vi "Inst_DS360.vi"(8 "error in":errorcluster, 10 "All Message Queues in":T1, 11 "Prueba09 in":refnum<class "Prueba09.lvclass">) -> (0 "error out":errorcluster)   [LabVIEW 2019, in "Prueba09.lvclass"]
uses:
  Prueba09.lvclass
  QMH/Message Queue/All Message Queues.ctl
  QMH/Message Queue/Message Cluster.ctl
  Prueba09.lvclass/Prueba09.ctl
  ClusterGEN.ctl
  <vilib>/Utility/error.llb/Error Cluster From Error Code.vi
  QMH/Message Queue/Enqueue Message (Single).vi
  <vilib>/ErrorRing/Error Ring.xnode
  QMH/Message Queue/Message Queue.lvlib
  Instrumento/DS360/DS360.lvclass
panel:
  out "All States":string[](array[string])
  out "Actual State":string
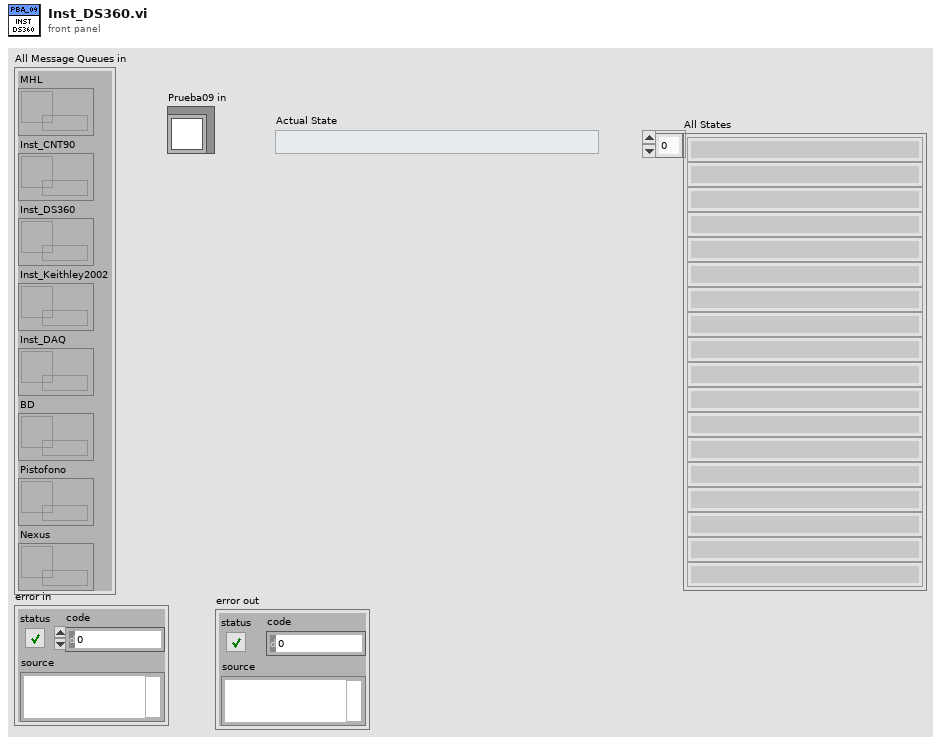
[diagram p1: front panel]
types:
  T1 = typedef "Message Queue.lvlib/All Message Queues.ctl" = cluster{"MHL":refnum<queue>, "Inst_CNT90":refnum<queue>, "Inst_DS360":refnum<queue>, "Inst_Keithley2002":refnum<queue>, "Inst_DAQ":refnum<queue>, "BD":refnum<queue>, "Pistofono":refnum<queue>, "Nexus":refnum<queue>}
  T2 = typedef "Prueba09.lvclass/ClusterGEN.ctl" = cluster{"frec":dbl, "amp":dbl, "tipo_ciclo":string}
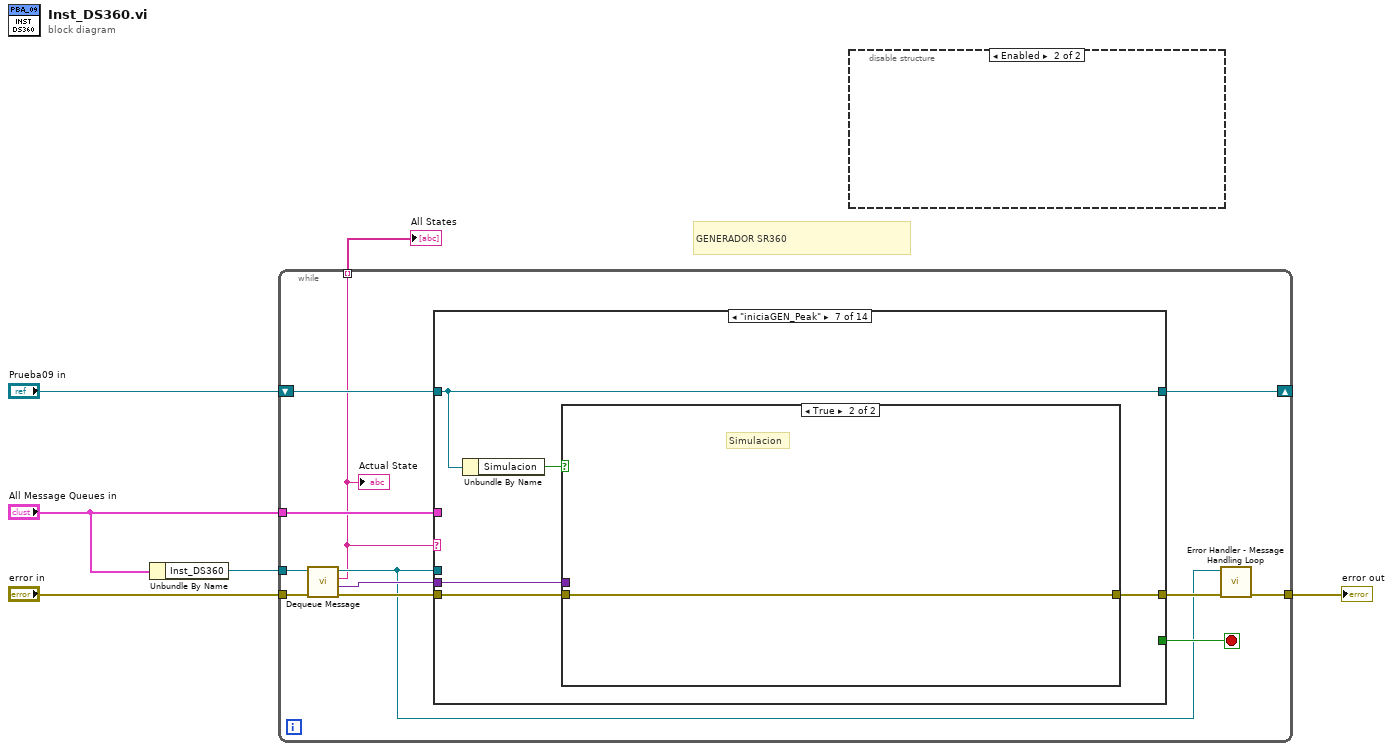
[diagram p0: block diagram]
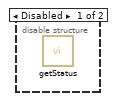
[diagram p2: hidden frame]
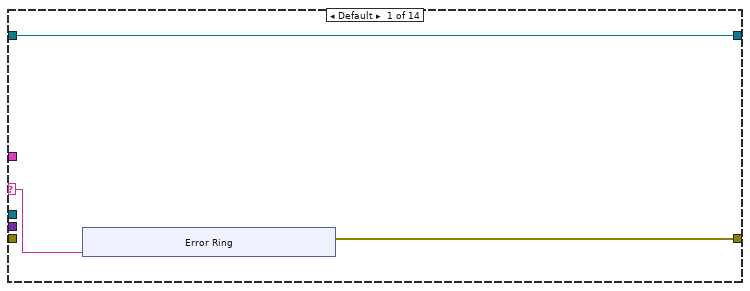
[diagram p3: hidden frame]
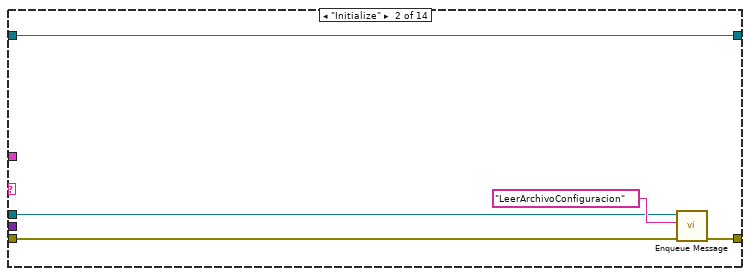
[diagram p4: hidden frame]
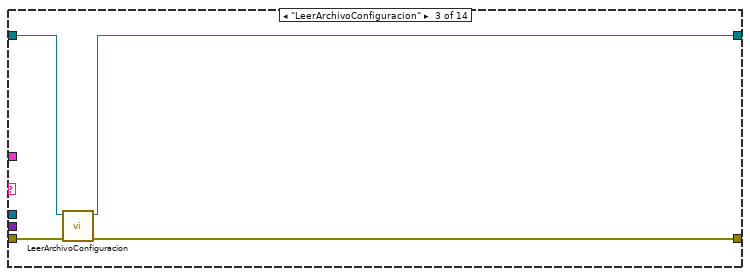
[diagram p5: hidden frame]
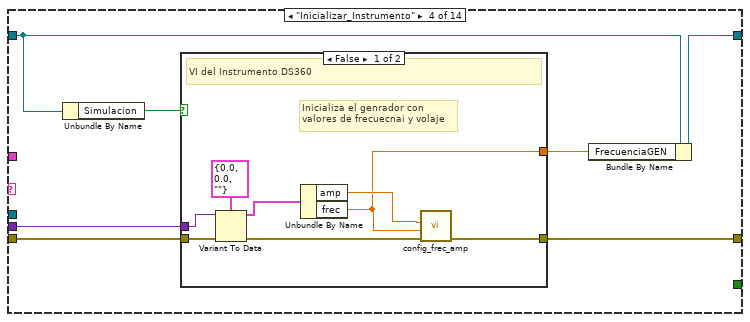
[diagram p6: hidden frame]
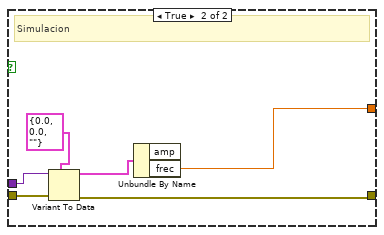
[diagram p7: hidden frame]
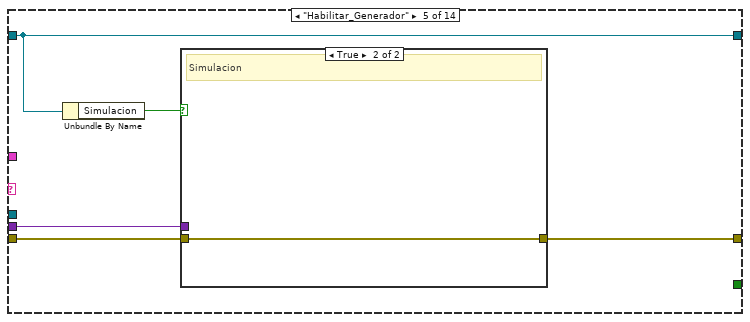
[diagram p8: hidden frame]
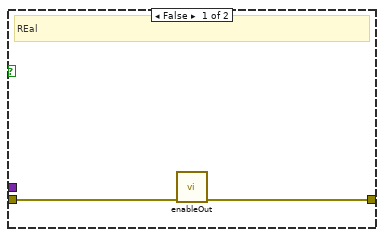
[diagram p9: hidden frame]
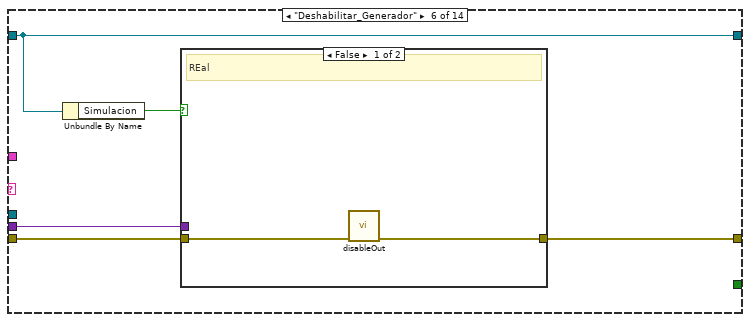
[diagram p10: hidden frame]
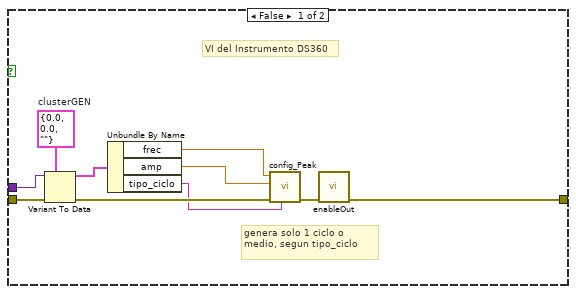
[diagram p12: hidden frame]
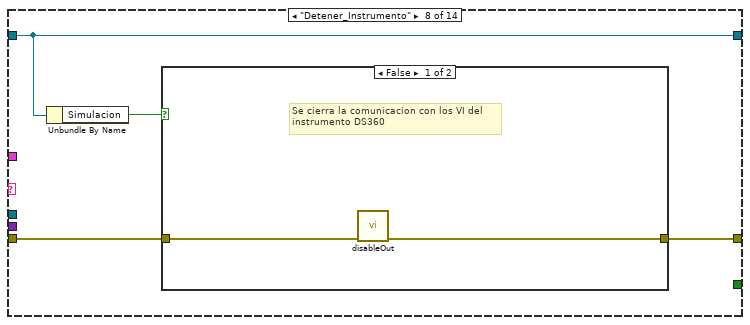
[diagram p13: hidden frame]
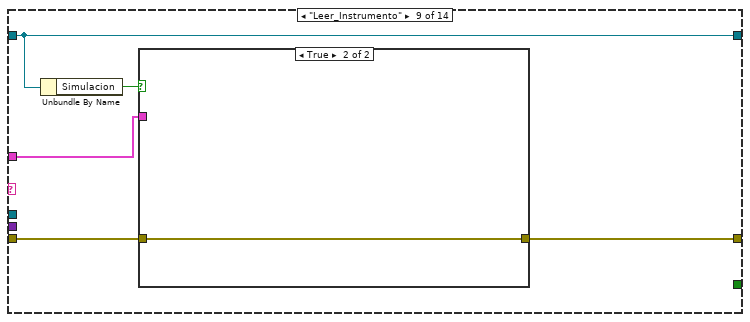
[diagram p15: hidden frame]
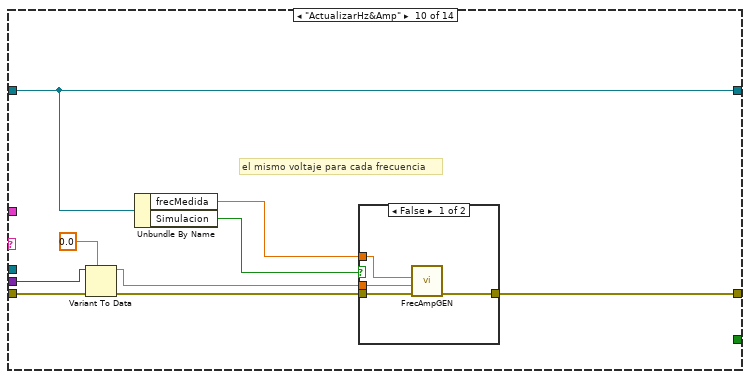
[diagram p17: hidden frame]
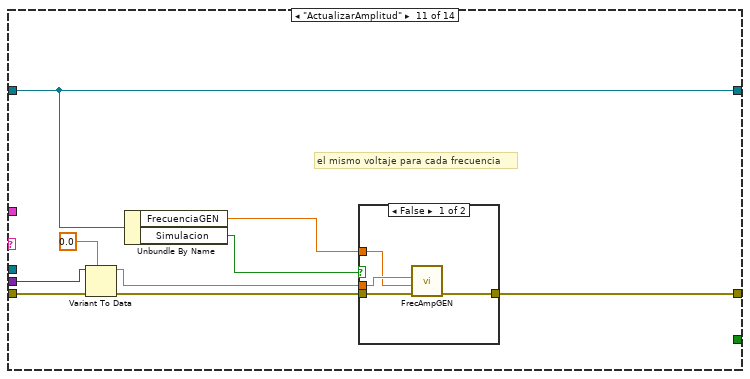
[diagram p19: hidden frame]
diagram:
  # "GENERADOR SR360"
  n1 = Unbundle By Name("All Message Queues in") -> ("Inst_DS360"=w4:refnum<queue>)
  n2 = while {
    tunnel: "error in" -> [w18]
    tunnel: w4 -> [w17]
    tunnel: "All Message Queues in" -> [w16]
    tunnel: [w9] -> w2
    shift-right: [w12] -> _
    shift-left: "Prueba09 in" -> [w15]
    tunnel: [w7] -> w1 mode=indexing
    stop <- w11 stop-if-true
    n3 = call "Dequeue Message.vi"("error in (no error)"=w18, "Message Queue"=w17) -> ("error out"=w13:errorcluster, "Message Data"=w14:variant, "Message"=w7:string, "dup Message Queue"=w8:refnum<queue>)  [unwired: 6 in]
    "Actual State" <- w7
    n4 = case shown="\"iniciaGEN_Peak\"" w7 {
      selector: w7 -> [w21 _ _ _ _ _ _ _ _ _ _ _ w147 _]
      tunnel: w16 -> [_ _ _ _ _ _ _ _ w101 _ _ _ w146 _]
      tunnel: w15 -> [w19 w33 w34 w42 w62 w70 w77 w93 w100 w109 w123 w136 w154 w156]
      tunnel: w8 -> [_ w29 _ _ _ _ _ _ _ _ _ _ _ w158]
      tunnel: w14 -> [_ _ _ w41 w61 w69 w76 _ _ w110 w124 w137 w151 _]
      tunnel: w13 -> [_ w30 w36 w40 w60 w68 w75 w91 w102 w111 w125 w138 w152 w159]
      tunnel: [w20 w31 w37 w44 w59 w67 w79 w94 w98 w113 w127 w140 w149 w155] -> w10
      tunnel: [w19 w33 w35 w39 w62 w70 w77 w93 w100 w109 w123 w136 w154 w156] -> w12
      tunnel: [_ _ _ _ _ _ _ _ _ _ _ _ _ TRUE] -> w11
      frame Default {
        n5 = xnode "Error Ring"("parameter 0"=w21) -> ("error out"=w20:errorcluster)
      }
      frame "Initialize" {
        n6 = call-poly "Enqueue Message.vi"("error in (no error)"=w30, "Message"="LeerArchivoConfiguracion", "Message Queue"=w29) -> ("error out"=w31:errorcluster)  [unwired: 7 in, 1 out]
      }
      frame "LeerArchivoConfiguracion" {
        n7 = call "LeerArchivoConfiguracion.vi"("error in"=w36, "Prueba31 in"=w34) -> ("error out"=w37:errorcluster, "Prueba31 out"=w35:refnum<class "Prueba09.lvclass">)  [unwired: 8 in]
      }
      frame "Inicializar_Instrumento" {
        n8 = Unbundle By Name(w42) -> ("Simulacion"=w43:bool)
        n9 = case shown="False" w43 {
          tunnel: [w51 w56] -> w44
          tunnel: w40 -> [w52 w58]
          tunnel: w41 -> [w49 w57]
          tunnel: [w46 w53] -> w38
          frame False {
            # "Inicializa el genrador con \nvalores de frecuecnai y volaje"
            # "VI del Instrumento DS360"
            n10 = Variant To Data(error in=w52, type=T2 {"frec"=0.0, "amp"=0.0, "tipo_ciclo"=""} ("clusterGEN"), Variant=w49) -> (data=w48:T2, error out=w50:errorcluster)
            n11 = Unbundle By Name(w48) -> ("amp"=w47:dbl, "frec"=w46:dbl)
            n12 = call "config_frec_amp.vi"("error in (no error)"=w50, "Frec (Hz)"=w46, "Amplitud (Vrms)"=w47) -> ("error out"=w51:errorcluster)  [unwired: 7 in, 1 out]
          }
          frame True {
            # "Simulacion"
            n13 = Variant To Data(error in=w58, type=T2 {"frec"=0.0, "amp"=0.0, "tipo_ciclo"=""} ("clusterGEN"), Variant=w57) -> (data=w54:T2, error out=w56:errorcluster)
            n14 = Unbundle By Name(w54) -> ("frec"=w53:dbl)  [unwired: 1 out]
          }
        }
        n15 = Bundle By Name(cluster=w42, "FrecuenciaGEN"=w38) -> (w39:refnum<class "Prueba09.lvclass">)
      }
      frame "Habilitar_Generador" {
        n16 = Unbundle By Name(w62) -> ("Simulacion"=w63:bool)
        n17 = case shown="True" w63 {
          tunnel: w60 -> [w65 w66]
          tunnel: w61 -> [_ _]
          tunnel: [w64 w66] -> w59
          frame False {
            # "REal"
            n18 = call "enableOut.vi"("error in (no error)"=w65) -> ("error out"=w64:errorcluster)  [unwired: 9 in, 1 out]
          }
          frame True {
            # "Simulacion"
          }
        }
      }
      frame "Deshabilitar_Generador" {
        n19 = Unbundle By Name(w70) -> ("Simulacion"=w71:bool)
        n20 = case shown="False" w71 {
          tunnel: w68 -> [w73 w74]
          tunnel: w69 -> [_ _]
          tunnel: [w72 w74] -> w67
          frame False {
            # "REal"
            n21 = call "disableOut.vi"("error in (no error)"=w73) -> ("error out"=w72:errorcluster)  [unwired: 9 in, 1 out]
          }
          frame True {
            # "Simulacion"
          }
        }
      }
      frame "iniciaGEN_Peak" {
        n22 = Unbundle By Name(w77) -> ("Simulacion"=w78:bool)
        n23 = case shown="True" w78 {
          tunnel: [w83 w90] -> w79
          tunnel: w75 -> [w89 w90]
          tunnel: w76 -> [w88 _]
          frame False {
            w86 = T2 {"frec"=0.0, "amp"=0.0, "tipo_ciclo"=""}  # clusterGEN
            # "genera solo 1 ciclo o medio, segun tipo_ciclo"
            # "VI del Instrumento DS360"
            n24 = Variant To Data(error in=w89, type=w86, Variant=w88) -> (data=w87:T2, error out=w84:errorcluster)
            n25 = Unbundle By Name(w87) -> ("frec"=w82:dbl, "amp"=w81:dbl, "tipo_ciclo"=w80:string)
            n26 = call "config_Peak.vi"("tipo_ciclo"=w80, "error in (no error)"=w84, "Amplitud (Vrms)"=w81, "Frec (Hz)"=w82) -> ("error out"=w85:errorcluster)  [unwired: 6 in, 1 out]
            n27 = call "enableOut.vi"("error in (no error)"=w85) -> ("error out"=w83:errorcluster)  [unwired: 9 in, 1 out]
          }
          frame True {
            # "Simulacion"
          }
        }
      }
      frame "Detener_Instrumento" {
        n28 = Unbundle By Name(w93) -> ("Simulacion"=w92:bool)
        n29 = case shown="False" w92 {
          tunnel: [w96 w97] -> w94
          tunnel: w91 -> [w95 w97]
          frame False {
            # "Se cierra la comunicacion con los VI del\ninstrumento DS360"
            n30 = call "disableOut.vi"("error in (no error)"=w95) -> ("error out"=w96:errorcluster)  [unwired: 9 in, 1 out]
          }
          frame True {
            # "Simulacion"
          }
        }
      }
      frame "Leer_Instrumento" {
        n31 = Unbundle By Name(w100) -> ("Simulacion"=w99:bool)
        n32 = case shown="True" w99 {
          tunnel: [w103 w104] -> w98
          tunnel: w102 -> [w103 w104]
          tunnel: w101 -> [_ _]
          frame False {
          }
          frame True {
          }
        }
      }
      frame "ActualizarHz&Amp" {
        # "el mismo voltaje para cada frecuencia"
        n33 = Variant To Data(error in=w111, type=0.0, Variant=w110) -> (data=w106:dbl, error out=w112:errorcluster)
        n34 = Unbundle By Name(w109) -> ("frecMedida"=w108:dbl, "Simulacion"=w105:bool)
        n35 = case shown="False" w105 {
          tunnel: [w117 w118] -> w113
          tunnel: w112 -> [w116 w118]
          tunnel: w108 -> [w115 _]
          tunnel: w106 -> [w114 _]
          frame False {
            n36 = call "FrecAmpGEN.vi"("error in (no error)"=w116, "Frec (Hz)"=w114, "Amplitud (Vrms)"=w115) -> ("error out"=w117:errorcluster)  [unwired: 7 in, 1 out]
          }
          frame True {
            # "Simlacion"
          }
        }
      }
      frame "ActualizarAmplitud" {
        # "el mismo voltaje para cada frecuencia"
        n37 = Variant To Data(error in=w125, type=0.0, Variant=w124) -> (data=w121:dbl, error out=w126:errorcluster)
        n38 = Unbundle By Name(w123) -> ("FrecuenciaGEN"=w119:dbl, "Simulacion"=w120:bool)
        n39 = case shown="False" w120 {
          tunnel: [w131 w132] -> w127
          tunnel: w126 -> [w130 w132]
          tunnel: w121 -> [w129 _]
          tunnel: w119 -> [w128 _]
          frame False {
            n40 = call "FrecAmpGEN.vi"("error in (no error)"=w130, "Frec (Hz)"=w128, "Amplitud (Vrms)"=w129) -> ("error out"=w131:errorcluster)  [unwired: 7 in, 1 out]
          }
          frame True {
            # "Simlacion"
          }
        }
      }
      frame "ActualizarFrecuencia" {
        # "el mismo voltaje para cada frecuencia"
        n41 = Variant To Data(error in=w138, type=0.0, Variant=w137) -> (data=w134:dbl, error out=w139:errorcluster)
        n42 = Unbundle By Name(w136) -> ("Simulacion"=w133:bool)
        n43 = case shown="False" w133 {
          tunnel: [w143 w144] -> w140
          tunnel: w139 -> [w142 w144]
          tunnel: w134 -> [w141 _]
          frame False {
            n44 = call "FrecAmpGEN.vi"("error in (no error)"=w142, "Frec (Hz)"=w141) -> ("error out"=w143:errorcluster)  [unwired: 8 in, 1 out]
          }
          frame True {
            # "Simlacion"
          }
        }
      }
      frame "Error" {
        n45 = Unbundle By Name(w146) -> ("MHL"=w145:refnum<queue>)
        n46 = Variant To Data(error in=w152, type=errorcluster {"status"=FALSE, "code"=0, "source"=""} ("error constant"), Variant=w151) -> (data=w148:errorcluster, error out=w150:errorcluster)
        n47 = call-poly "Enqueue Message.vi"("error in (no error)"=w150, "Message Data"=w148, "Message"=w147, "Message Queue"=w145) -> ("error out"=w149:errorcluster)  [unwired: 6 in, 1 out]
      }
      frame "Exit" {
        n48 = Release Queue(queue=w158, error in (no error)=w159) -> (error out=w155:errorcluster)  [unwired: 1 in, 2 out]
      }
    }
    n49 = call "Error Handler - Message Handling Loop.vi"("error in (no error)"=w10, "Message Queue"=w8) -> ("dup error in"=w9:errorcluster)  [unwired: 8 in, 1 out]
  }
  "error out" <- w2
  "All States" <- w1
  n50 = disable-structure shown="Enabled" {
    frame Disabled {
      n51 = call "getStatus.vi"() -> ()  [unwired: 9 in, 3 out]
    }
    frame Enabled {
    }
  }
